vi "lab7_task1.vi"() -> ()   [LabVIEW 2021]
uses:
  <vilib>/Analysis/NI_AALBase.lvlib
  <vilib>/Analysis/1siggen.llb/Ramp Pattern by Samples.vi
  <vilib>/DAQmx/write.llb/DAQmx Write (Analog DBL 1Chan 1Samp).vi
  <vilib>/DAQmx/read.llb/DAQmx Read (Analog DBL 1Chan 1Samp).vi
panel:
  out "XY Graph":cluster{"X":dbl, "Y":dbl}[](graph)
  in  "start":dbl format="%0.2f"
  in  "end":dbl=1.0 format="%0.2f"
  in  "samples":i32=128
  out "# Sample":i32
  out "Voltage Output":dbl
  in  "stop":bool
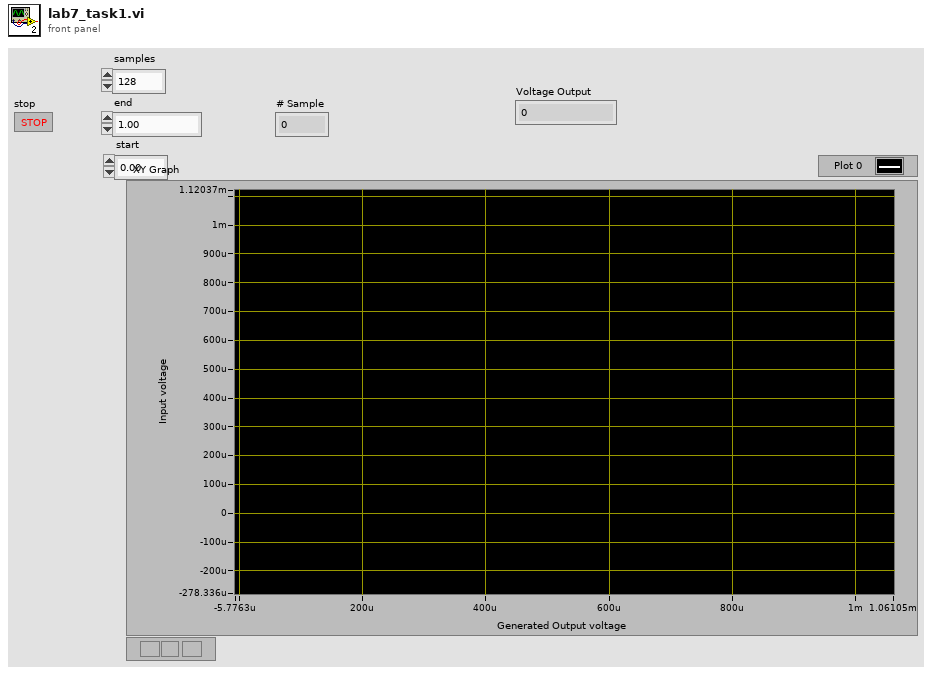
[diagram p1: front panel]
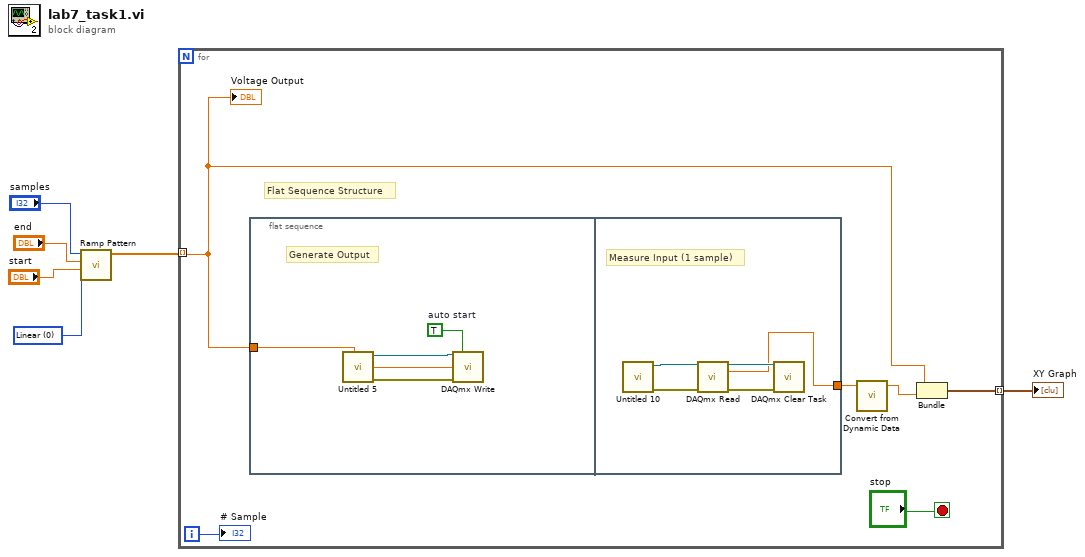
[diagram p0: block diagram]
diagram:
  w3 = u16 0 items=["Linear", "Logarithmic"] ("type")
  n1 = call-poly <vilib>:"Ramp Pattern.vi"("type"=w3, "start"="start", "end"="end", "samples"="samples") -> ("Ramp Pattern"=w2:dbl[])  [unwired: 6 in, 1 out]
  n2 = for {
    tunnel: w2 -> [w10] mode=indexing
    tunnel: [w8] -> w1 mode=indexing
    i -> [w12]
    stop <- "stop" stop-if-true
    # "Flat Sequence Structure"
    n3 = flat-sequence {
      tunnel: w10 -> [w13]
      tunnel: [w17] -> w7
      frame #0 {
        w16 = TRUE  # auto start
        # "Generate Output"
        n4 = call "Untitled 5.vi"() -> ("error out"=w14:errorcluster, "task out"=w15:refnum<k21>)  [unwired: 10 in]
        n5 = call-poly <vilib>:"DAQmx Write.vi"("task/channels in"=w15, "auto start"=w16, "data"=w13, "error in"=w14) -> ()  [unwired: 9 in, 3 out]
      }
      frame #1 {
        # "Measure Input (1 sample)"
        n6 = call "Untitled 10.vi"() -> ("error out"=w18:errorcluster, "task out"=w19:refnum<k21>)  [unwired: 10 in]
        n7 = call-poly <vilib>:"DAQmx Read.vi"("task/channels in"=w19, "error in"=w18) -> ("task out"=w20:refnum<k21>, "data"=w17:dbl, "error out"=w21:errorcluster)  [unwired: 11 in]
        n8 = call <vilib>:"DAQmx Clear Task.vi"("task in"=w20, "error in"=w21) -> ()  [unwired: 13 in, 1 out]
      }
    }
    n9 = call "Convert from Dynamic Data"("Dynamic Data Type"=w7) -> ("Scalar"=w11:dbl)  [unwired: 3 in]
    n10 = Bundle(w10, "Scalar"=w11) -> (w8:cluster{dbl, "Scalar":dbl})  [unwired: 1 in]
    "# Sample" <- w12
    "Voltage Output" <- w10
  }
  "XY Graph" <- w1
